vi "Last Modified Cache.vi"(7 "Allow Shared Cache? (F)":bool, 8 "error in (no error)":errorcluster, 9 "Max Age":i32, 10 "Last Modified":timestamp, 11 "Response in":refnum<class "Response.lvclass">) -> (0 "error out":errorcluster, 3 "Response out":refnum<class "Response.lvclass">)   [LabVIEW 2020, in "HTTP Utils.lvlib" / "Response.lvclass"]
uses:
  Response.lvclass
  Response.lvclass/Response.ctl
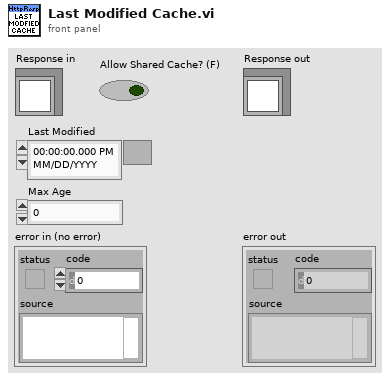
[diagram p1: front panel]
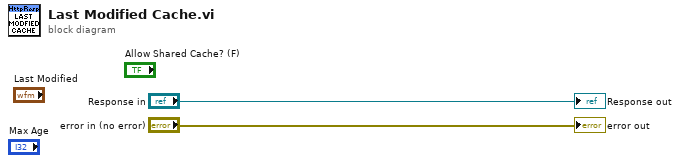
[diagram p0: block diagram]
diagram:
  "error out" <- "error in (no error)"
  "Response out" <- "Response in"
